vi "calibrateEvent.vi"(8 "error in (no error)":errorcluster, 11 "RampEvent in":refnum<class "RampEvent.lvclass">) -> (0 "error out":errorcluster, 3 "RampEvent out":refnum<class "RampEvent.lvclass">)   [LabVIEW 2009, in "Tools.lvlib" / "Scripting.lvlib" / "RampEvent.lvclass"]
uses:
  RampEvent.lvclass
  ScriptEvent.lvclass
  RampEvent.lvclass/RampEvent.ctl
  DatabaseHelpers/Database Objects/Channel/Channel.lvclass
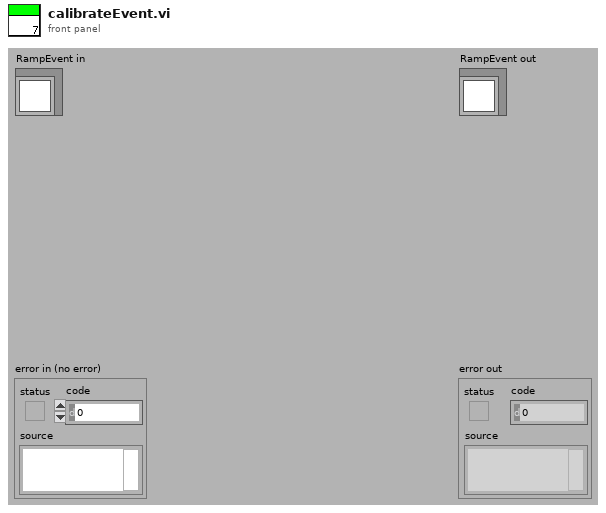
[diagram p1: front panel]
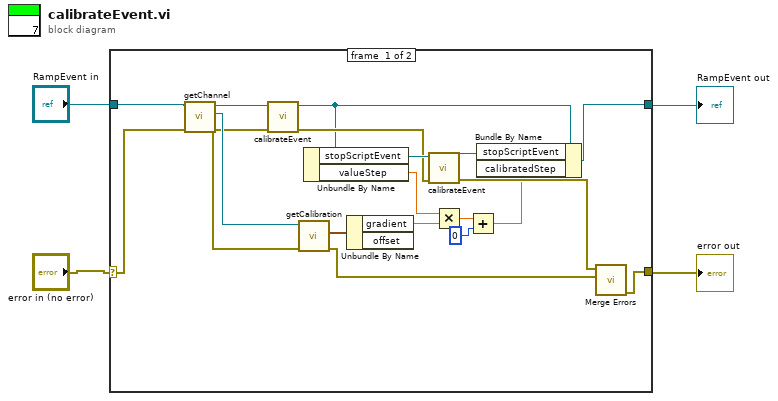
[diagram p0: block diagram]
diagram:
  n1 = case shown="No Error" "error in (no error)" {
    selector: "error in (no error)" -> [w11 w24]
    tunnel: [w6 w24] -> w4
    tunnel: [w19 w25] -> w3
    tunnel: "RampEvent in" -> [w12 w25]
    frame #0 {
      n2 = call-dynamic "getChannel.vi"("error in (no error)"=w11, "ScriptEvent.lvclass in"=w12) -> ("error out"=w9:errorcluster, "Channel.lvclass"=w10:refnum<class "Channel.lvclass">, "ScriptEvent.lvclass out"=w13:refnum<class "RampEvent.lvclass">)  [unwired: 7 in]
      n3 = call-parent "calibrateEvent.vi"("error in (no error)"=w9, "ScriptEvent in"=w13) -> ("error out"=w22:errorcluster, "ScriptEvent out"=w20:refnum<class "RampEvent.lvclass">)  [unwired: 8 in]
      n4 = call "getCalibration.vi"("error in (no error)"=w9, "Channel.lvclass in"=w10) -> ("error out"=w15:errorcluster, "calibration"=w18:cluster{"gradient":dbl, "offset":dbl})  [unwired: 7 in, 1 out]
      n5 = Unbundle By Name(w20) -> ("stopScriptEvent"=w23:refnum<class "ScriptEvent.lvclass">, "valueStep"=w14:dbl)
      n6 = Unbundle By Name(w18) -> ("gradient"=w17:dbl)  [unwired: 1 out]
      n7 = call-parent "calibrateEvent.vi"("error in (no error)"=w22, "ScriptEvent in"=w23) -> ("error out"=w8:errorcluster, "ScriptEvent out"=w21:refnum<class "ScriptEvent.lvclass">)  [unwired: 8 in]
      n8 = Multiply(x=w14, y=w17) -> (x*y=w16:dbl)
      n9 = Add(x=w16, y=0) -> (x+y=w7:dbl)
      n10 = Bundle By Name(cluster=w20, "stopScriptEvent"=w21, "calibratedStep"=w7) -> (w19:refnum<class "RampEvent.lvclass">)
      n11 = call <vilib>:"Merge Errors.vi"("error in 2 (no error)"=w15, "error in 1 (no error)"=w8) -> ("error out"=w6:errorcluster)  [unwired: 5 in]
    }
    frame #1 {
    }
  }
  "error out" <- w4
  "RampEvent out" <- w3
